vi "Temperatura.vi"() -> ()   [LabVIEW 2010]
uses:
  <vilib>/express/express analysis/Spectral/XNode/ExpressSpectralMeasurementsBlockNode.xnode
  <vilib>/express/express analysis/Spectral/Block/exnSpectralBlock spectral measurements RMS poly.vi
  <vilib>/express/express analysis/Spectral/Block/exnSpectralBlock spectral measurements RMS DDT.vi
  <vilib>/Analysis/NI_AALBase.lvlib
panel:
  out "Filtro+media":dbl format="%#_4g"
  out "Media":dbl format="%#_4g"
  out "Waveform Graph 3":dynamicdata(graph)
  out "Waveform Chart":dynamicdata(graph)
  out "Waveform Graph 2":dynamicdata(graph)
  out "Real":dbl
  out "Waveform Graph":dynamicdata(graph)
  in  "stop":bool
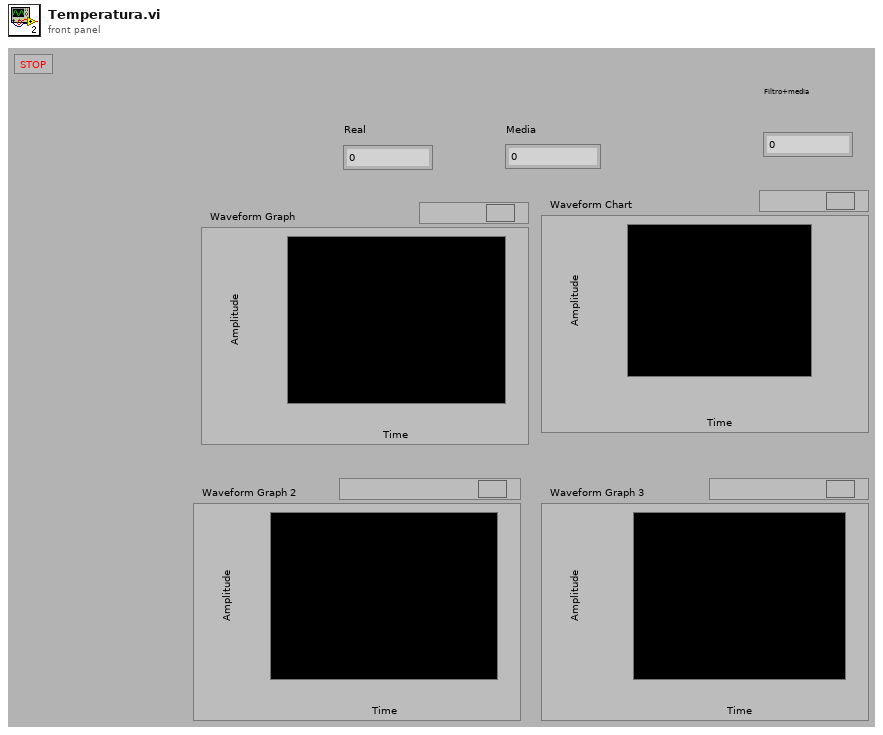
[diagram p1: front panel]
types:
  T1 = cluster{"averaging mode":u16, "weighting mode":u16, "number of averages":u32}
  T2 = cluster{"dB On (F)":bool, "unwrap phase (F)":bool, "convert to degree (F)":bool}
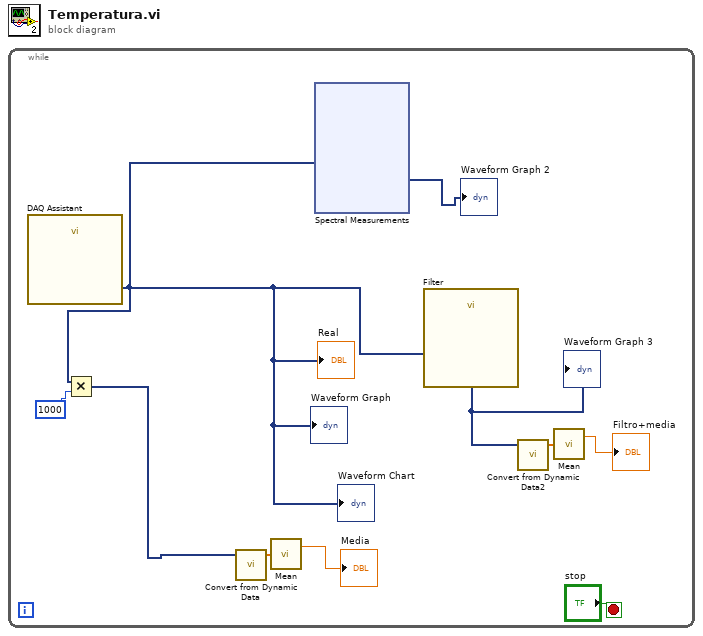
[diagram p0: block diagram]
diagram:
  n1 = while {
    stop <- "stop" stop-if-true
    n2 = call "DAQ Assistant"() -> ("data"=w3:dynamicdata)  [unwired: 17 in, 2 out]
    "Waveform Graph" <- w3
    "Real" <- w3
    "Waveform Chart" <- w3
    n3 = Multiply(x=w3, y=1000) -> (x*y=w1:dynamicdata)
    n4 = call "Convert from Dynamic Data"("Dynamic Data Type"=w1) -> ("Array"=w8:dbl[])  [unwired: 3 in]
    n5 = call <vilib>:"Mean.vi"("X"=w8) -> ("mean"=→"Media":dbl)  [unwired: 1 out]
    n6 = xnode "Spectral Measurements"("Signals"=w3) -> ("FFT - (RMS)"=→"Waveform Graph 2":dynamicdata)  [unwired: 1 in, 2 out]
    n7 = call "Filter"("Signal"=w3) -> ("Filtered Signal"=w6:dynamicdata)  [unwired: 9 in, 1 out]
    "Waveform Graph 3" <- w6
    n8 = call "Convert from Dynamic Data2"("Dynamic Data Type"=w6) -> ("Array"=w5:dbl[])  [unwired: 3 in]
    n9 = call <vilib>:"Mean.vi"("X"=w5) -> ("mean"=→"Filtro+media":dbl)  [unwired: 1 out]
  }
